vi "Set Test No and Parameters.vi"(3 "Channel Select":T1(ring), 6 "Test Parameters In":refnum<vi>) -> (0 "Test Parameters Out":T2 {"Rx Channel" min=1 max=1024; "Tx Channel" min=1 max=1024})   [LabVIEW 2026]
uses:
  <instrlib>/MicroPulse/Public/Data/Datatypes/MP - test parameters.ctl
  <instrlib>/MicroPulse/MicroPulse_Driver.lvlib
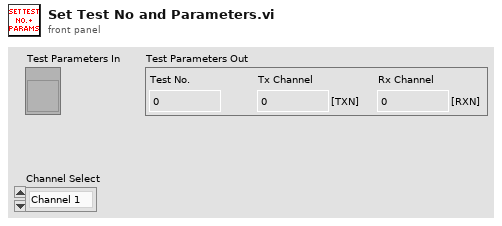
[diagram p1: front panel]
types:
  T1 = enum16{"Channel 1", "Channel 2", "Channel 3", "Channel 4", "Channel 5", "Channel 6", "Channel 7"}
  T2 = typedef "MicroPulse_Driver.lvlib/MP - test parameters.ctl" = cluster{"Test No.":u32, "Tx Channel":u32, "Rx Channel":u32}
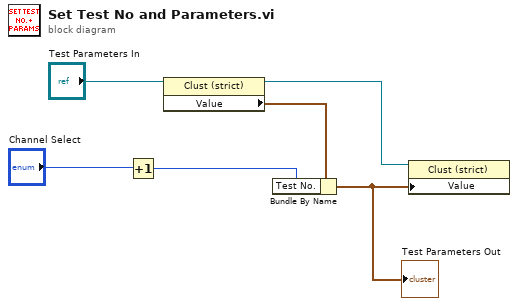
[diagram p0: block diagram]
diagram:
  n1 = Increment(x="Channel Select") -> (x+1=w4:T1)
  n2 = property class="Clust (strict)"(reference="Test Parameters In") -> (reference out=w5:refnum<vi>, "Value"=w2:T2)  [unwired: 1 in, 1 out]
  n3 = Bundle By Name(cluster=w2, "Test No."=w4) -> (w6:T2)
  "Test Parameters Out" <- w6
  n4 = property class="Clust (strict)"(reference=w5, "Value"=w6) -> ()  [unwired: 1 in, 2 out]
